vi "Tracker_v2_test_acq_comms_channel.vi"() -> ()   [LabVIEW 2018]
uses:
  <vilib>/Instr/_visa.llb/Select Event Type.ctl
  <vilib>/Platform/TimedLoop/XDataNode/timing_clust.ctl
  <vilib>/Platform/TimedLoop/XDataNode/nitl_modes.ctl
  <vilib>/Platform/TimedLoop/XDataNode/wakeup.ctl
  <extravilib>/ChannelInstances/High Speed Stream-c(str,stamp)/_Read For Replicate.vi
  <vilib>/Platform/TimedLoop/scheduler/LVUserAPI/_suppVIs/Create_1kHz_TSource.vi
  <extravilib>/ChannelInstances/High Speed Stream-c(str,stamp)/Instantiate.vi
  <extravilib>/ChannelInstances/High Speed Stream-c(str,stamp)/)Channel.vi
  <extravilib>/ChannelInstances/High Speed Stream-c(str,stamp)/Abort Signal/Init Signal.vi
  <vilib>/Platform/TimedLoop/XDataNode/XDataNode.xnode
  Tracker.lvlib
  <vilib>/Analysis/NI_AALBase.lvlib
  <extravilib>/ChannelInstances/High Speed Stream-c(str,stamp).lvlib
  <vilib>/Platform/TimedLoop/XDataNode/XDNodeRunTimeDep.lvlib
panel:
  out "standard deviation":dbl format="%0.3f"
  out "mean frame time, ms":dbl format="%0.3f"
  out "count":i32
  out "Instrument OK?":bool=TRUE
  out "Data frame channel sink":T1
  out "Data frame channel source":T2
  in  "Play/Pause":bool
  in  "Stop Button":bool
  in  "VISA resource name in":refnum<visa-resource-name>="ASRL3::INSTR"
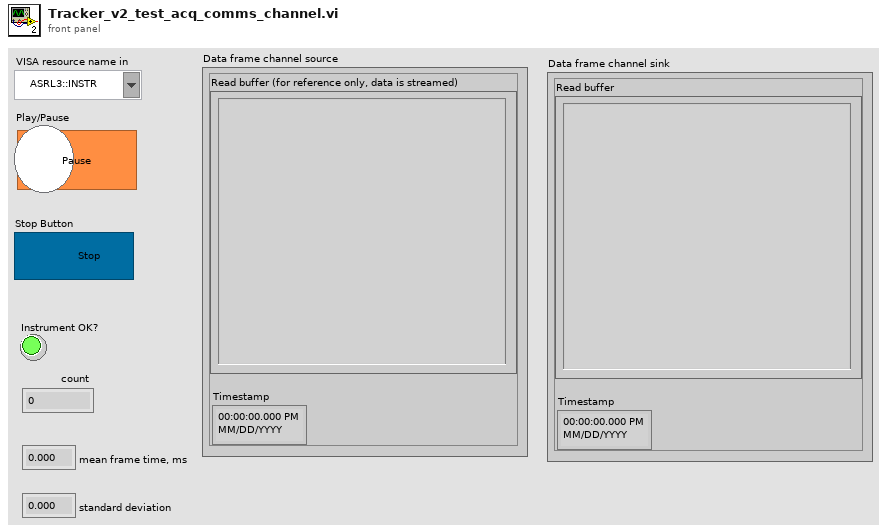
[diagram p1: front panel]
types:
  T1 = cluster{"Read buffer":string, "Timestamp":timestamp}
  T2 = cluster{"Read buffer (for reference only, data is streamed)":string, "Timestamp":timestamp}
  T3 = typedef "Select Event Type.ctl" = u32
  T4 = typedef "Tracker.lvlib/CTL_Data_flow_control_cluster.ctl" = cluster{"Data acquisition status":refnum<notifier>, "Play/Pause status":refnum<notifier>, "Complete stop":refnum<notifier>, "Temp file ready for processing":refnum<notifier>, "Has been recorded":refnum<notifier>, "Recording now":refnum<notifier>, "Path to the latest complete temp file":refnum<notifier>, "(Final) Data file is saved":refnum<notifier>, "Data loaded":refnum<notifier>}
  T5 = typedef "XDNodeRunTimeDep.lvlib/timing_clust.ctl" = cluster{"Expected End [f-1]":u64, "Actual End [f-1]":u64, "Finished Late? [f-1]":bool, "Expected End [i-1]":u64, "Actual End [i-1]":u64, "Finished Late? [i-1]":bool, "Expected Start [i]":u64, "Actual Start [i]":u64, "Expected Start [f]":u64, "Actual Start [f]":u64, "Source Name":string, "Structure Name":string, "Period":i64, "Deadline":i64, "Offset":i64, "Start":i64, "Priority":i32, "Timeout":i32, "Mode":T6, "Wakeup Reason":T7, "Error":errorcluster, "Source Type":string, "Secondary Source Type":string, "Global End Time":u64, "Global Start Time":u64, "Frame Duration":u64, "Iteration Duration":u64, "Assigned CPU":i32, "I/O Scan Engine Mode":u32}
  T6 = typedef "XDNodeRunTimeDep.lvlib/nitl_modes.ctl" = enum32{"No Change", "Process missed periods, maintain original phase", "Discard missed periods, maintain original phase", "Process missed periods, ignore original phase", "Discard missed periods, ignore original phase"}
  T7 = typedef "XDNodeRunTimeDep.lvlib/wakeup.ctl" = enum32{"Normal", "Aborted", "Asynchronous wakeup", "Timing source error", "Timed loop error", "Timeout"}
  T8 = typedef "High Speed Stream-c(str,stamp).lvlib/)Channel.ctl" = refnum<queue>
  T9 = cluster{"Data acquisition status":refnum<notifier>, "Play/Pause status":refnum<notifier>, "Complete stop":refnum<notifier>, "Temp file ready for processing":refnum<notifier>, "Has been recorded":refnum<notifier>, "Recording now":refnum<notifier>, "Path to the latest complete temp file":refnum<notifier>, "Final CSV saved":refnum<notifier>, "Data loaded":refnum<notifier>}
  T10 = cluster{"Read buffer (for reference only, data is queued)":string, "Timestamp":timestamp}
  T11 = cluster{string, "seconds since 1Jan1904":timestamp}
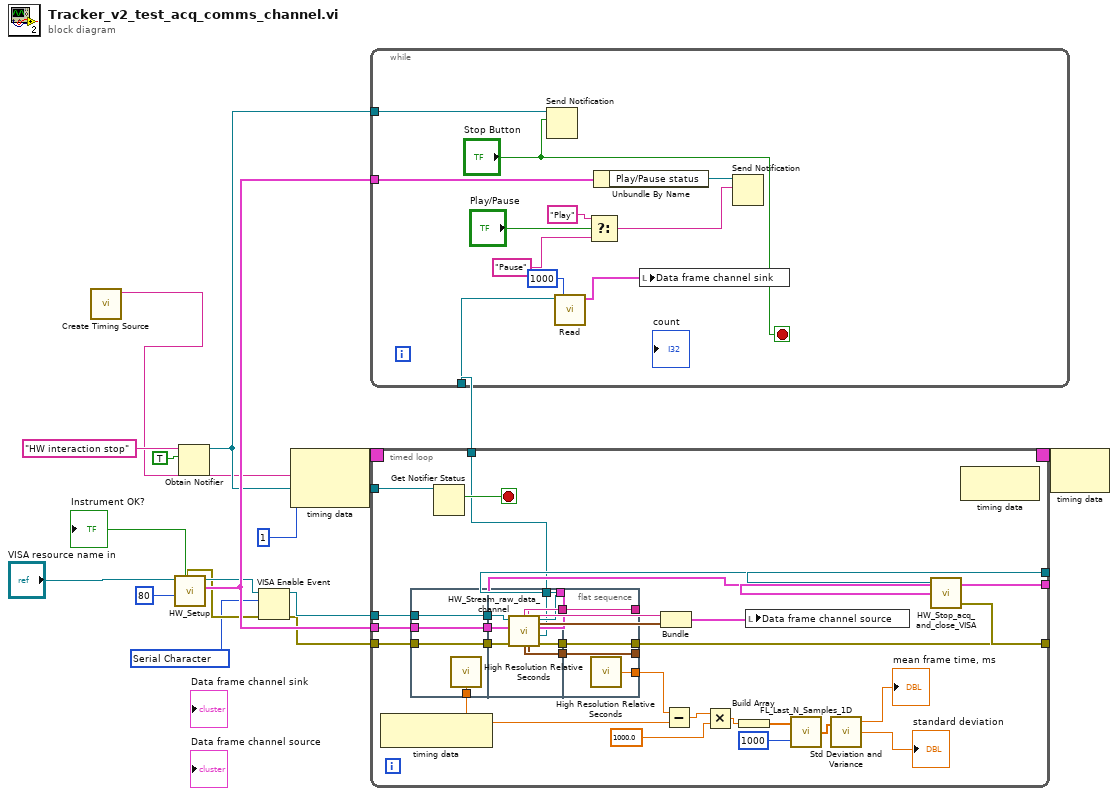
[diagram p0: block diagram]
diagram:
  w3 = T3 1073684533 items=["Service Request"=1073684491, "Trigger"=3221168138, "Clear"=1073684493, "VXI Signal"=1073684512, "VXI/VME Interrupt"=3221168161, "VXI/VME Sysfail"=1073684509, "VXI/VME Sysreset"=1073684510, "GPIB CIC"=1073684498, "GPIB Talk"=1073684499, "GPIB Listen"=1073684500, "PXI Interrupt"=1073684514, "Serial Break"=1073684515, "Serial TermChar"=1073684516, "Serial CTS"=1073684521, "Serial DSR"=1073684522, "Serial DCD"=1073684524, "Serial RI"=1073684526, "Serial Character"=1073684533, "USB Interrupt"=1073684535, "All Enabled"=1073709055] ("Event Type")
  n1 = call-poly <vilib>:"Create Timing Source.vi"() -> ("name (out)"=w10:string)  [unwired: 10 in, 1 out]
  n2 = call "HW_Setup.vi"("Traget FPS"=80, "VISA resource name in"="VISA resource name in") -> ("Instrument OK?"=→"Instrument OK?":bool, "Data flow controls"=w18:T4, "VISA resource name out"=w7:refnum<visa-resource-name>, "error out"=w5:errorcluster)  [unwired: 2 in, 4 out]
  n3 = Obtain Notifier(name (unnamed)="HW interaction stop", notification data type=TRUE) -> (notifier out=w15:refnum<notifier>)  [unwired: 2 in, 2 out]
  n4 = VISA Enable Event(8:w5, 10:w3, 11:w7) -> (0:w4:errorcluster, 3:w6:refnum<visa-resource-name>)  [unwired: 1 in]
  n5 = node-c288(w10, i64 1 ("Period")) -> (w12:T5)
  n6 = timed-loop {
    tunnel: w6 -> [w48]
    tunnel: [w45] -> w1
    tunnel: w18 -> [w47]
    tunnel: [w44] -> w19
    tunnel: w4 -> [w46]
    tunnel: [w41] -> w2
    tunnel: w15 -> [w43]
    tunnel: [w38] -> w14
    timing: w12 -> [_]
    timing-out: [_] -> w11
    stop <- w42 stop-if-true
    n7 = node-c288() -> ()  [unwired: 1 in, 1 out]
    n8 = flat-sequence {
      tunnel: w46 -> [w52]
      tunnel: w47 -> [w53]
      tunnel: w48 -> [w54]
      tunnel: [w54] -> w37
      tunnel: [w53] -> w36
      tunnel: [w52] -> w35
      tunnel: [w51] -> w30
      tunnel: [w60] -> w45
      tunnel: [w59] -> w44
      tunnel: [w55] -> w38
      tunnel: w37 -> [w63]
      tunnel: w36 -> [w62]
      tunnel: w35 -> [w61]
      tunnel: [w58] -> w34
      tunnel: [w57] -> w33
      tunnel: [w56] -> w32
      tunnel: [w65] -> w39
      tunnel: [w66] -> w40
      tunnel: [w67] -> w41
      tunnel: w34 -> [w67]
      tunnel: w33 -> [w66]
      tunnel: w32 -> [w65]
      tunnel: [w64] -> w31
      frame #0 {
        n9 = call <vilib>:"High Resolution Relative Seconds.vi"() -> ("relative seconds"=w51:dbl)
      }
      frame #1 {
        n10 = call "HW_Stream_raw_data_channel.vi"("error in"=w61, "Data flow controls in"=w62, "VISA resource name in"=w63) -> ("error out"=w58:errorcluster, "High-speed channel"=w55:T8, "Data flow controls out"=w59:T9, "VISA resource name out"=w60:refnum<visa-resource-name>, "Timestamp"=w56:timestamp, "Read buffer (for reference only, data is queued)"=w57:string)  [unwired: 3 in]
      }
      frame #2 {
        n11 = call <vilib>:"High Resolution Relative Seconds.vi"() -> ("relative seconds"=w64:dbl)
      }
    }
    n12 = Get Notifier Status(notifier=w43) -> (current notification=w42:bool)  [unwired: 1 in, 4 out]
    n13 = Bundle("Read buffer (for reference only, data is queued)"=w40, "Timestamp"=w39) -> (w21:T10)  [unwired: 1 in]
    n14 = Subtract(x=w31, y=w30) -> (x-y=w29:dbl)
    n15 = Multiply(x=w29, y=1000.0) -> (x*y=w22:dbl)
    n16 = Build Array(w22) -> (w27:dbl[])
    n17 = local write "Data frame channel source"(w21) -> ()
    n18 = call "FL_Last_N_Samples_1D.vi"("BufferLengthSamples"=u32 1000, "Input Array"=w27) -> ("Output Array"=w26:dbl[])
    n19 = call <vilib>:"Std Deviation and Variance.vi"("X"=w26) -> ("mean"=→"mean frame time, ms":dbl, "standard deviation"=→"standard deviation":dbl)  [unwired: 1 in, 1 out]
    n20 = node-c288() -> ()  [unwired: 1 in, 1 out]
  }
  n21 = while {
    tunnel: w18 -> [w78]
    tunnel: w15 -> [w72]
    tunnel: w14 -> [w70]
    stop <- "Stop Button" stop-if-true
    n22 = Send Notification(notification="Stop Button", notifier=w72) -> ()  [unwired: 1 in, 2 out]
    n23 = call <extravilib>:"Read.vi"("timeout in ms (-1)"=1000, "channel"=w70) -> ("element"=w68:T11)  [unwired: 5 in, 4 out]
    n24 = Select(t="Play", s="Play/Pause", f="Pause") -> (s? t:f=w75:string)
    n25 = Unbundle By Name(w78) -> ("Play/Pause status"=w77:refnum<notifier>)
    n26 = local write "Data frame channel sink"(w68) -> ()
    n27 = Send Notification(notification=w75, notifier=w77) -> ()  [unwired: 1 in, 2 out]
  }
  n28 = call "HW_Stop_acq_and_close_VISA.vi"("error in"=w2, "Data flow controls in"=w19, "VISA resource name in"=w1) -> ()  [unwired: 2 out]
  n29 = node-c288(w11) -> ()  [unwired: 1 out]
